vi "Charger_Is IPG Present.vi"(8 "error in":errorcluster, 11 "Status Refnum":T1) -> (0 "error out":errorcluster, 2 "IPG Present?":bool, 3 "Status Refnum OUT":T1)   [LabVIEW 2020]
uses:
  Charger_Status Refnum.ctl
  Drivers/Charger Test Set/Charger_Input Control.ctl
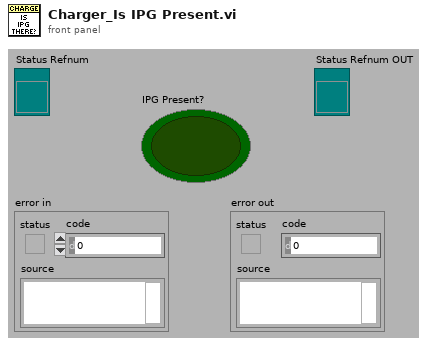
[diagram p1: front panel]
types:
  T1 = typedef "Charger_Status Refnum.ctl" = refnum<vi>
  T2 = typedef "Charger_Input Control.ctl" = cluster{"address":refnum<visa-resource-name>, "position":i32, "setpoint":dbl}
  T3 = cluster{"MICS ID":u32, "VBAT":dbl, "ChargingState":string, "VBAT Slide":dbl, "Status":string, "TemperatureLevel":dbl, "IPG_ReceivedLevel":dbl, "VBAT Target":dbl, "Charger Setpoint":dbl, "Index":i32, "Ready":bool, "Charger Inputs":T2, "MICS Inputs":cluster{"address":refnum<visa-resource-name>, "chan":u16, "ID":u32}}
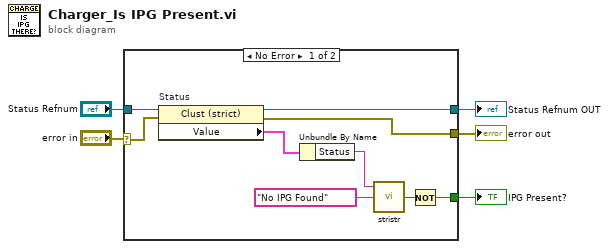
[diagram p0: block diagram]
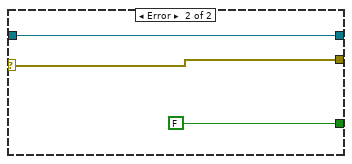
[diagram p2: hidden frame]
diagram:
  n1 = case shown="No Error" "error in" {
    selector: "error in" -> [w10 w17]
    tunnel: "Status Refnum" -> [w14 w16]
    tunnel: [w7 FALSE] -> w2
    tunnel: [w9 w16] -> w3
    tunnel: [w6 w17] -> w1
    frame No Error {
      n2 = property on="Status" class="Clust (strict)"(reference=w14, error in=w10) -> (reference out=w9:T1, error out=w6:errorcluster, "Value"=w13:T3)
      n3 = Unbundle By Name(w13) -> ("Status"=w11:string)
      n4 = call "stristr.vi"("Substring"="No IPG Found" ("regular expression"), "Input String"=w11) -> ("found"=w8:bool)  [unwired: 1 in, 2 out]
      n5 = Not(x=w8) -> (.not. x?=w7:bool)
    }
    frame Error {
    }
  }
  "Status Refnum OUT" <- w3
  "IPG Present?" <- w2
  "error out" <- w1
